vi "System_Write TagBus_deleteME.vi"(10 "TagBus.lvclass":refnum<class "TagBus.lvclass">, 11 "System in":refnum<class "System.lvclass">) -> (3 "System out":refnum<class "System.lvclass">)   [LabVIEW 2015]
uses:
  System.lvclass
  TagBus/TagBus.lvclass
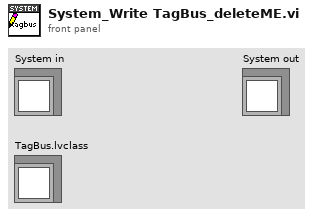
[diagram p1: front panel]
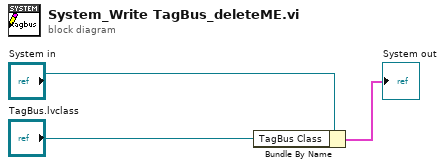
[diagram p0: block diagram]
diagram:
  n1 = Bundle By Name(cluster="System in", "TagBus Class"="TagBus.lvclass") -> (→"System out":cluster{})
